vi "BRig_Host__Loop_Consumer_RunState__typeTrial__subtypeEnd_parse.vi"(11 "input_strCmd":string) -> (2 "output_nTrial":u16)   [LabVIEW 2014]
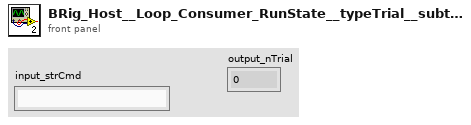
[diagram p1: front panel]
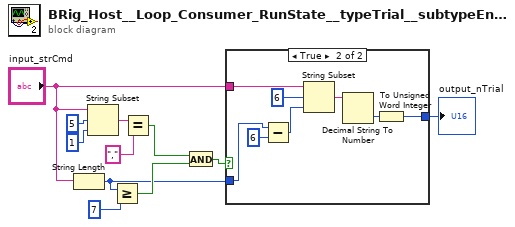
[diagram p0: block diagram]
diagram:
  n1 = String Length(string="input_strCmd") -> (length=w2:i32)
  n2 = String Subset(string="input_strCmd", offset (0)=5, length (rest)=1 ("offset (0)")) -> (substring=w9:string)
  n3 = Greater Or Equal?(x=w2, y=7) -> (x >= y?=w6:bool)
  n4 = Equal?(x=w9, y=",") -> (x = y?=w5:bool)
  n5 = And(x=w5, y=w6) -> (x .and. y?=w4:bool)
  n6 = case shown="True" w4 {
    tunnel: "input_strCmd" -> [_ w19]
    tunnel: w2 -> [_ w16]
    tunnel: [_ w12] -> w1
    frame False {
    }
    frame True {
      n7 = Subtract(x=w16, y=6) -> (x-y=w15:i32)
      n8 = String Subset(string=w19, offset (0)=6, length (rest)=w15) -> (substring=w14:string)
      n9 = Decimal String To Number(string=w14) -> (number=w13:i32)  [unwired: 2 in, 1 out]
      n10 = To Unsigned Word Integer(number=w13) -> (unsigned 16bit integer=w12:u16)
    }
  }
  "output_nTrial" <- w1
